vi "Test Worker Process Job Broadcasts Status.vi"(8 "error in (no error)":errorcluster, 11 "Worker Test in":refnum<class "Worker Test.lvclass">) -> (0 "error out":errorcluster, 3 "Worker Test out":refnum<class "Worker Test.lvclass">)   [LabVIEW 2020, in "Worker Test.lvclass"]
uses:
  Worker Test.lvclass
  C:/Program Files (x86)/National Instruments/LabVIEW 2020/vi.lib/Asteme/LUnit/Test Case.lvclass
  Worker/Worker.lvclass
  C:/Program Files (x86)/National Instruments/LabVIEW 2020/vi.lib/Asteme/Triarc Framework/Process/Process.lvclass
  <vilib>/Asteme/Triarc Framework/Process/Process.lvclass/Process.ctl
  <vilib>/Asteme/LUnit/Test Case.lvclass/Test Case.ctl
  <vilib>/Asteme/LUnit/LUnit Assertion Result.lvclass/LUnit Assertion Result.ctl
  <vilib>/Asteme/Triarc Framework Test Suite/Support/Execution timer.vi
  <vilib>/Asteme/Triarc Framework/Process/Private/SubVIs/Wait for finish.vi
  <vilib>/Asteme/Triarc Framework/Process/Protected/Messaging/Enqueue Message.vi
  <vilib>/Asteme/Triarc Framework/Process/Private/SubVIs/Set Lifecycle State.vi
  <vilib>/Asteme/Triarc Framework/Process/Public/Lifecycle/Get Lifecycle State.vi
  <vilib>/Asteme/LUnit/Palette/Pass If.vi
  <vilib>/Asteme/LUnit/Set Assertion Type.vi
  <vilib>/Asteme/LUnit/Add test result.vi
  <vilib>/Asteme/LUnit/LUnit Get Test Case.vi
  <vilib>/Asteme/LUnit/Assertion Result/LUnit Get Test Name.vi
  <vilib>/Asteme/LUnit/LUnit Write Message.vi
  <vilib>/Asteme/LUnit/LUnit Write Description.vi
  <vilib>/Asteme/LUnit/LUnit Write Skipped.vi
  <vilib>/Utility/error.llb/Clear Errors.vi
  <vilib>/Asteme/LUnit/Palette/Fail.vi
  <vilib>/Asteme/LUnit/Palette/Pass.vi
  <vilib>/Asteme/LUnit/LUnit Write Assertion Type.vi
  <vilib>/Asteme/LUnit/Read Test Case Name.vi
  <vilib>/Asteme/LUnit/LUnit Write Passed.vi
  <vilib>/Asteme/Triarc Framework Test Suite/Support/Event Helpers/Dequeue Event Message.vi
  <vilib>/Utility/error.llb/Error Cluster From Error Code.vi
  <vilib>/Asteme/LUnit/LUnit Assertion Result.lvclass
  <vilib>/Asteme/Triarc Framework/Process/Process.lvclass
  <vilib>/Asteme/Triarc Framework Test Suite/Support/Event Helpers/Event Helpers.lvlib
  <vilib>/Asteme/LUnit/Test Case.lvclass
  C:/Users/anton/Documents/GitHub/Triarc-Examples/Coffee Shop/Person/Person.lvclass
  C:/Program Files (x86)/National Instruments/LabVIEW 2020/vi.lib/Asteme/Triarc Framework/View/View.lvclass
  C:/Program Files (x86)/National Instruments/LabVIEW 2020/vi.lib/Asteme/Triarc Framework/Base/Base.lvclass
  C:/Program Files (x86)/National Instruments/LabVIEW 2020/vi.lib/Asteme/Triarc Framework/Error Handler Interface/Error Handler Interface.lvclass
  C:/Program Files (x86)/National Instruments/LabVIEW 2020/vi.lib/Asteme/Triarc Framework/Logging/Logging.lvclass
  C:/Users/anton/Documents/GitHub/Triarc-Examples/Coffee Shop/Worker/Worker.lvclass
  C:/Users/anton/Documents/GitHub/Triarc-Examples/Coffee Shop/Person Test/Person Test.lvclass
  C:/Program Files (x86)/National Instruments/LabVIEW 2020/vi.lib/Asteme/Triarc Framework Test Suite/View Test/View Test.lvclass
  C:/Program Files (x86)/National Instruments/LabVIEW 2020/vi.lib/Asteme/Triarc Framework Test Suite/Process Test/Process Test.lvclass
  C:/Program Files (x86)/National Instruments/LabVIEW 2020/vi.lib/Asteme/Triarc Framework Test Suite/Base Class Test/Base Test.lvclass
  C:/Users/anton/Documents/GitHub/Triarc-Examples/Coffee Shop/Worker Test/Worker Test.lvclass
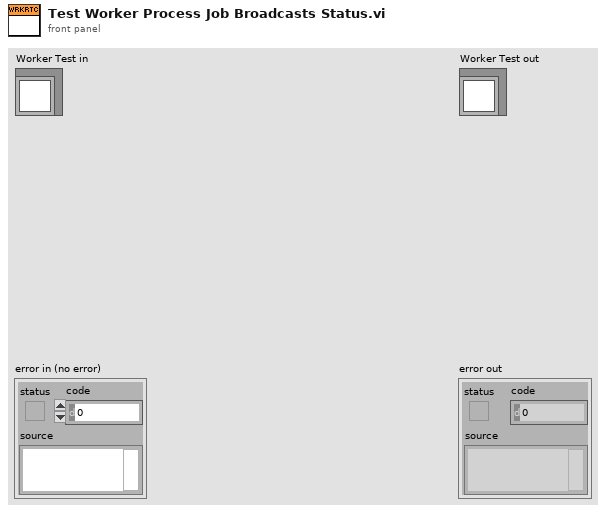
[diagram p1: front panel]
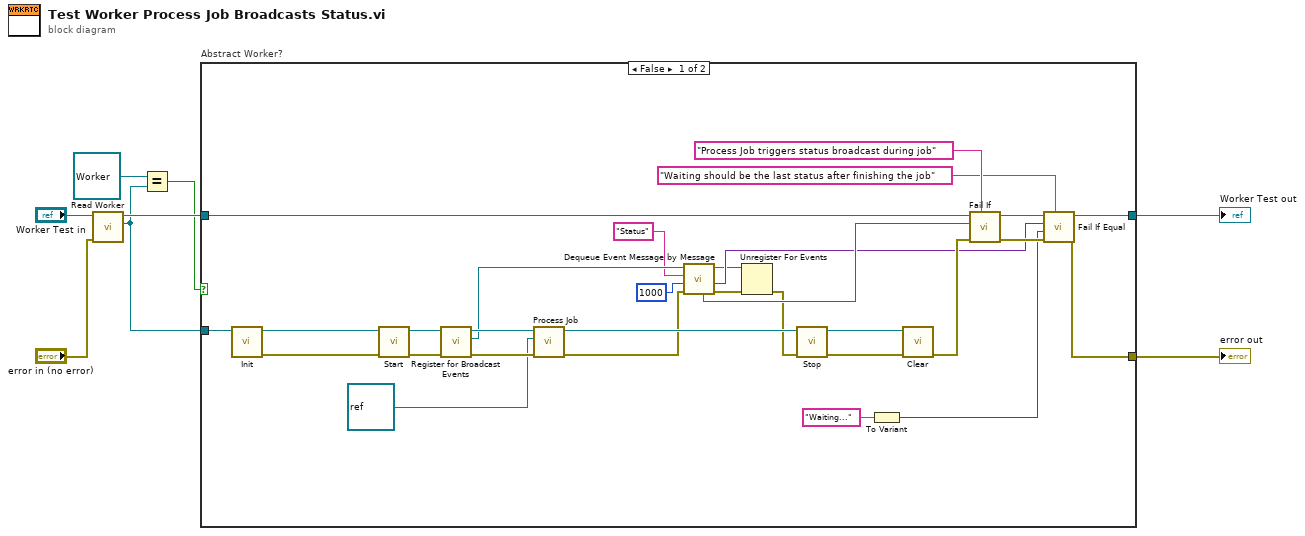
[diagram p0: block diagram]
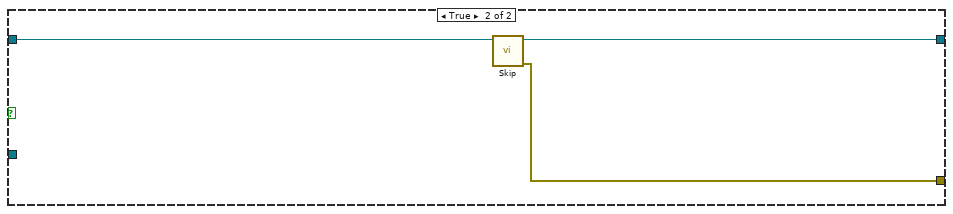
[diagram p2: hidden frame]
diagram:
  n1 = call "Read Worker.vi"("error in (no error)"="error in (no error)", "Worker Test in"="Worker Test in") -> ("Worker"=w2:refnum<class "Worker.lvclass">, "Worker Test out"=w5:refnum<class "Worker Test.lvclass">)  [unwired: 7 in, 1 out]
  n2 = Equal?(x=refnum<class "Worker.lvclass"> refnum ("Worker"), y=w2) -> (x = y?=w1:bool)
  n3 = case "Abstract Worker?" shown="False" w1 {
    tunnel: [w17 w39] -> w6
    tunnel: w5 -> [w31 w41]
    tunnel: [w15 w40] -> w4
    tunnel: w2 -> [w19 _]
    frame False {
      n4 = call-dynamic "Init.vi"("View In"=w19) -> ("error out"=w38:errorcluster, "View Out"=w35:refnum<class "Worker.lvclass">)  [unwired: 9 in]
      n5 = call <vilib>:"Start.vi"("error in (no error)"=w38, "Process In"=w35) -> ("error out"=w34:errorcluster, "Process Out"=w28:refnum<class "Worker.lvclass">)  [unwired: 8 in]
      n6 = call <vilib>:"Register for Broadcast Events.vi"("error in (no error)"=w34, "Process In"=w28) -> ("error out"=w29:errorcluster, "Event Registration Refnum Out"=w23:refnum<event-registration>, "Process Out"=w27:refnum<class "Worker.lvclass">)  [unwired: 7 in]
      n7 = call "Process Job.vi"("error in (no error)"=w29, "Task"=refnum<class> refnum, "Worker In"=w27) -> ("error out"=w25:errorcluster, "Worker Out"=w26:refnum<class "Worker.lvclass">)  [unwired: 7 in]
      n8 = call <vilib>:"Dequeue Event Message by Message.vi"("error in (no error)"=w25, "Timeout (-1)"=1000, "Message"="Status", "Event Registration Refnum"=w23) -> ("error out"=w20:errorcluster, "Message Data"=w14:variant, "Event Registration Refnum Out"=w9:refnum<event-registration>, "Timed Out?"=w18:bool)  [unwired: 3 in, 1 out]
      n9 = Unregister For Events(event registration refnum=w9, error in=w20) -> (error out=w10:errorcluster)
      n10 = call <vilib>:"Stop.vi"("error in (no error)"=w10, "Process In"=w26) -> ("error out"=w36:errorcluster, "Process Out"=w37:refnum<class "Worker.lvclass">)  [unwired: 7 in, 1 out]
      n11 = To Variant(anything="Waiting...") -> (Variant=w12:variant)
      n12 = call-dynamic "Clear.vi"("error in (no error)"=w36, "View In"=w37) -> ("error out"=w33:errorcluster)  [unwired: 9 in]
      n13 = call <vilib>:"Fail If.vi"("Description"="Process Job triggers status broadcast during job", "error in (no error)"=w33, "Fail?"=w18, "Test Case In"=w31) -> ("error out"=w32:errorcluster, "Test Case Out"=w16:refnum<class "Worker Test.lvclass">)  [unwired: 6 in]
      n14 = call <vilib>:"Fail If Equal.vi"("Description"="Waiting should be the last status after finishing the job", "error in (no error)"=w32, "Actual"=w12, "Expected"=w14, "Test Case In"=w16) -> ("error out"=w17:errorcluster, "Test Case Out"=w15:refnum<class "Worker Test.lvclass">)  [unwired: 5 in]
    }
    frame True {
      n15 = call <vilib>:"Skip.vi"("Test Case In"=w41) -> ("error out"=w39:errorcluster, "Test Case Out"=w40:refnum<class "Worker Test.lvclass">)  [unwired: 9 in]
    }
  }
  "error out" <- w6
  "Worker Test out" <- w4
